vi "Server.vi"() -> ()   [LabVIEW 2013]
panel:
  in  "port":u16=31180
  in  "service name":string="127.0.0.1"
  in  "DCV":dbl format="%.9f"
  in  "Status":string="measuring"
  in  "Result":string
  out "CMD":string
  in  "Stop":bool
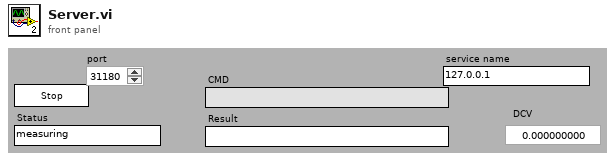
[diagram p1: front panel]
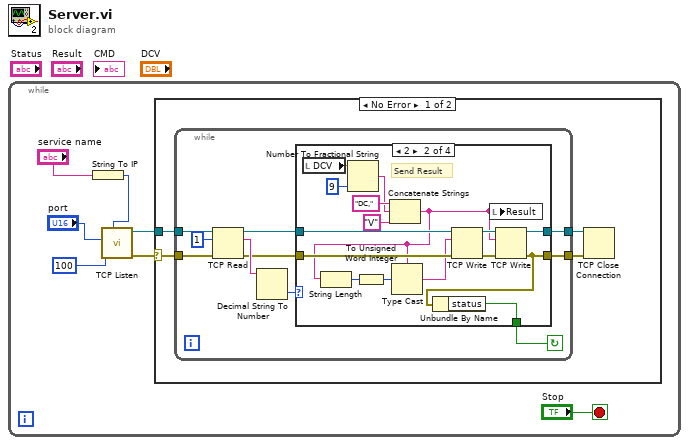
[diagram p0: block diagram]
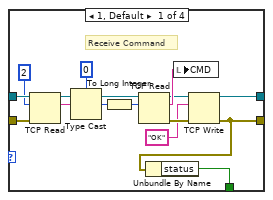
[diagram p2: hidden frame]
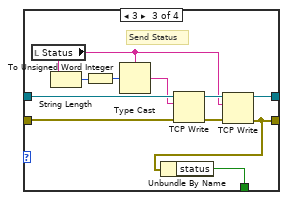
[diagram p3: hidden frame]
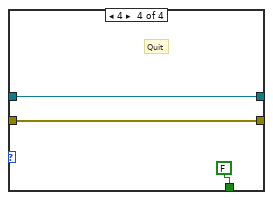
[diagram p4: hidden frame]
diagram:
  n1 = while {
    stop <- "Stop" stop-if-true
    n2 = String To IP(1:"service name") -> (0:w1:u32)
    n3 = call <vilib>:"TCP Listen.vi"("net address"=w1, "timeout ms (wait forever: -1)"=100, "port"="port") -> ("error out"=w6:errorcluster, "connection ID"=w4:refnum<k5>)  [unwired: 4 in, 3 out]
    n4 = case shown="No Error" w6 {
      selector: w6 -> [w10 _]
      tunnel: w4 -> [w11 _]
      frame No Error {
        n5 = while {
          tunnel: w11 -> [w21]
          tunnel: w10 -> [w20]
          tunnel: [w14] -> w9
          tunnel: [w13] -> w8
          stop <- w16 continue-if-true
          n6 = TCP Read(connection ID=w21, bytes to read=1, error in (no error)=w20) -> (connection ID out=w15:refnum<k5>, data out=w18:string, error out=w12:errorcluster)  [unwired: 2 in]
          n7 = Decimal String To Number(string=w18) -> (number=w17:i32)  [unwired: 2 in, 1 out]
          n8 = case shown="2" w17 {
            tunnel: [w35 w52 w63 FALSE ("status")] -> w16
            tunnel: w15 -> [w29 w41 w60 w66]
            tunnel: [w31 w51 w62 w66] -> w14
            tunnel: [w30 w50 w61 w65] -> w13
            tunnel: w12 -> [w28 w42 w59 w65]
            frame 1, Default {
              # "Receive Command"
              n9 = TCP Read(connection ID=w29, bytes to read=2, error in (no error)=w28) -> (connection ID out=w26:refnum<k5>, data out=w25:string)  [unwired: 2 in, 1 out]
              n10 = Type Cast(type=u16 0 ("bytes to read"), x=w25) -> (*(type *) &x=w24:u16)
              n11 = To Long Integer(number=w24) -> (32bit integer=w22:i32)
              n12 = TCP Read(connection ID=w26, bytes to read=w22) -> (connection ID out=w34:refnum<k5>, data out=w36:string, error out=w33:errorcluster)  [unwired: 3 in]
              n13 = local write "CMD"(w36) -> ()
              n14 = TCP Write(connection ID=w34, data in="OK", error in (no error)=w33) -> (connection ID out=w31:refnum<k5>, error out=w30:errorcluster)  [unwired: 1 in, 1 out]
              n15 = Unbundle By Name(w30) -> ("status"=w35:bool)
            }
            frame 2 {
              # "Send Result"
              n16 = local read "DCV"() -> (w49:dbl)
              n17 = Number To Fractional String(number=w49, precision (6)=i16 9) -> (F-format string=w46:string)  [unwired: 2 in]
              n18 = Concatenate Strings("DC," ("string"), w46, "V" ("string")) -> (w37:string)
              n19 = String Length(string=w37) -> (length=w40:i32)
              n20 = To Unsigned Word Integer(number=w40) -> (unsigned 16bit integer=w39:u16)
              n21 = Type Cast(type=w37, x=w39) -> (*(type *) &x=w38:string)
              n22 = TCP Write(connection ID=w41, data in=w38, error in (no error)=w42) -> (connection ID out=w43:refnum<k5>, error out=w44:errorcluster)  [unwired: 1 in, 1 out]
              n23 = local write "Result"(w37) -> ()
              n24 = TCP Write(connection ID=w43, data in=w37, error in (no error)=w44) -> (connection ID out=w51:refnum<k5>, error out=w50:errorcluster)  [unwired: 1 in, 1 out]
              n25 = Unbundle By Name(w50) -> ("status"=w52:bool)
            }
            frame 3 {
              # "Send Status"
              n26 = local read "Status"() -> (w54:string)
              n27 = String Length(string=w54) -> (length=w56:i32)
              n28 = To Unsigned Word Integer(number=w56) -> (unsigned 16bit integer=w55:u16)
              n29 = Type Cast(type=w54, x=w55) -> (*(type *) &x=w53:string)
              n30 = TCP Write(connection ID=w60, data in=w53, error in (no error)=w59) -> (connection ID out=w57:refnum<k5>, error out=w58:errorcluster)  [unwired: 1 in, 1 out]
              n31 = TCP Write(connection ID=w57, data in=w54, error in (no error)=w58) -> (connection ID out=w62:refnum<k5>, error out=w61:errorcluster)  [unwired: 1 in, 1 out]
              n32 = Unbundle By Name(w61) -> ("status"=w63:bool)
            }
            frame 4 {
              # "Quit"
            }
          }
        }
        n33 = TCP Close Connection(connection ID=w9, error in (no error)=w8) -> ()  [unwired: 1 in, 2 out]
      }
      frame Error {
      }
    }
  }
